vi "生成word报表.vi"(0 "Array输入":refnum<vi>, 1 "产品序号":string, 2 "标注图":T1(plugin-control), 3 "Array输入 2":refnum<vi>, 4 "测试人":string, 5 "部位":string, 8 "反射图":T1(plugin-control) caption="Original Image") -> (14 "报告生成路径":path)   [LabVIEW 2018]
uses:
  <vilib>/Utility/NIReport.llb/Report Type.ctl
  <vilib>/Utility/NIReport.llb/Append Report Text (str wrap).vi
  <vilib>/addons/_office/word.llb/Word Edit Cell ([dbl]).vi
  <vilib>/addons/_office/word.llb/Word Edit Cell (str).vi
  <vilib>/Utility/NIReport.llb/Append Report Text (num wrap).vi
  <vilib>/Utility/NIReport.llb/NI_report.lvclass
  <vilib>/addons/_office/NI_ReportGenerationToolkit.lvlib
  <vilib>/Utility/NIReport.llb/Word/NI_Word.lvclass
  <vilib>/Utility/NIReport.llb/NI_ReportGenerationCore.lvlib
  <vilib>/addons/_office/word.llb/Word Edit Cell ([str]).vi
panel:
  out "分层累计缺陷占比":dbl
  out "分层Z值":dbl[](array[numeric])
  out "缺陷个数 2":i32
  out "分层数据":dbl[][](array[numeric])
  out "弥散累计缺陷占比":dbl
  out "弥散数据":dbl[][](array[numeric])
  out "弥散Z值":dbl[](array[numeric])
  out "缺陷个数":i32
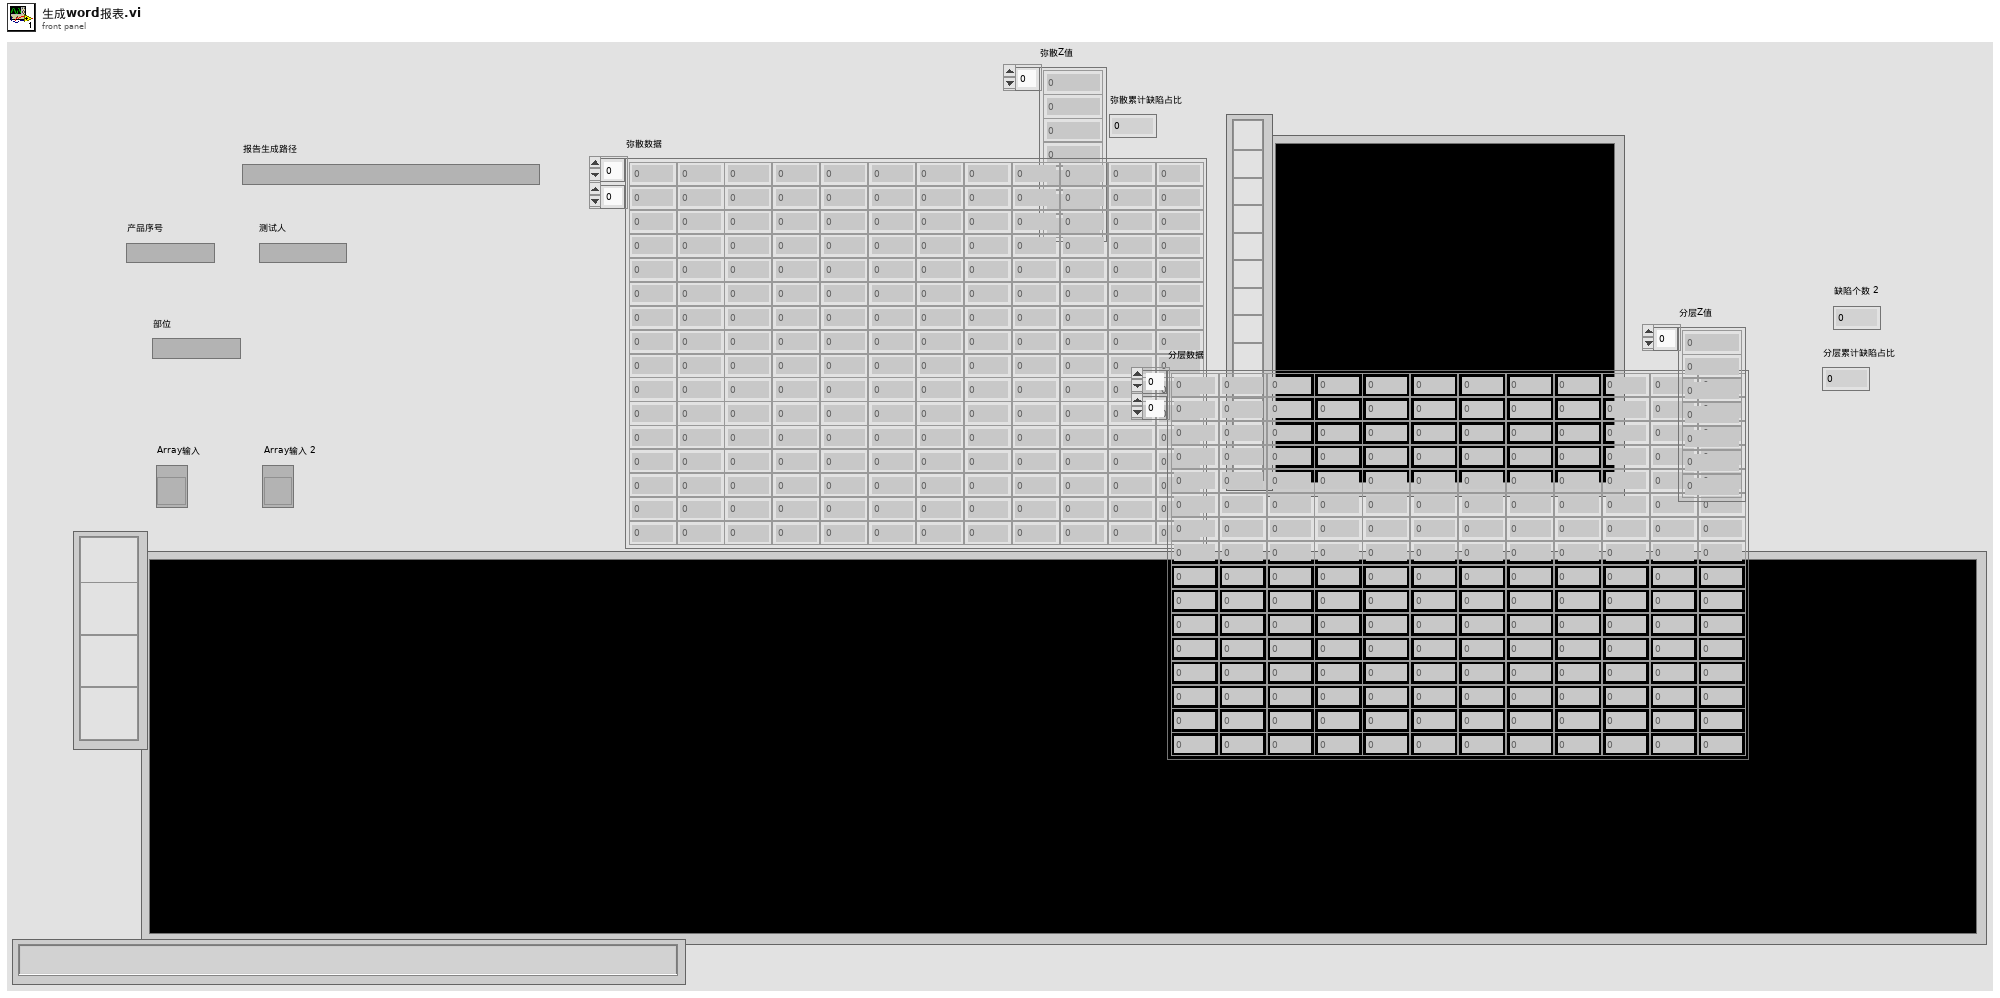
[diagram p1: front panel]
types:
  T1 = typedef "IMAQ Image.ctl" = refnum<image>
  T2 = cluster{"position (Excel)":cluster{"row":i32, "column":i32}, "name (Excel)":string, "bookmark (Word)":string}
  T3 = typedef "NI_ReportGenerationCore.lvlib/Report Type.ctl" = enum16{"HTML", "Word", "Excel"}
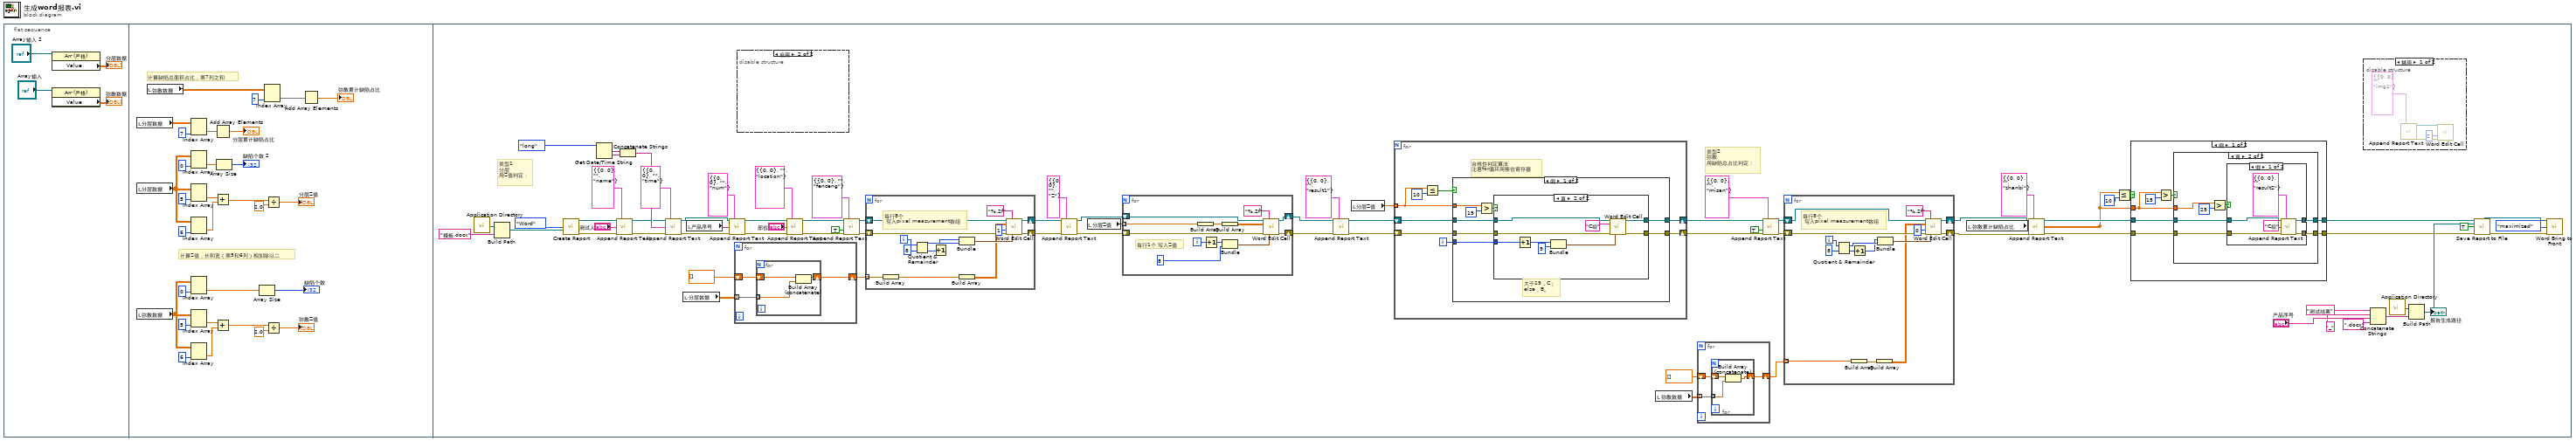
[diagram p0: block diagram]
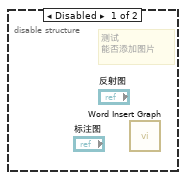
[diagram p3: hidden frame]
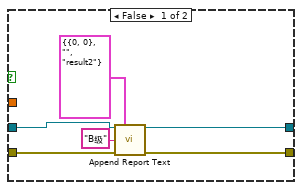
[diagram p4: hidden frame]
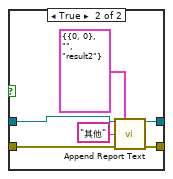
[diagram p5: hidden frame]
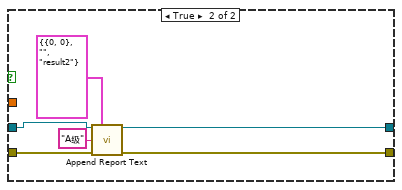
[diagram p6: hidden frame]
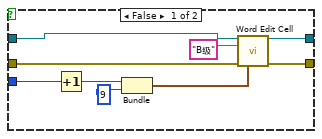
[diagram p7: hidden frame]
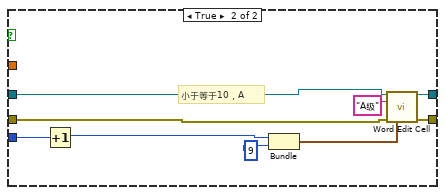
[diagram p8: hidden frame]
diagram:
  n1 = flat-sequence {
    frame #0 {
      n2 = property class="Arr (严格)"(reference="Array输入 2") -> ("Value"=→"分层数据":dbl[][])  [unwired: 1 in, 2 out]
      n3 = property class="Arr (严格)"(reference="Array输入") -> ("Value"=→"弥散数据":dbl[][])  [unwired: 1 in, 2 out]
    }
    frame #1 {
      # "计算缺陷总面积占比，第7列之和"
      # "计算Z值，长和宽（第5和6列）相加除以二"
      n4 = local read "分层数据"() -> (w8:dbl[][])
      n5 = local read "分层数据"() -> (w19:dbl[][])
      n6 = local read "弥散数据"() -> (w34:dbl[][])
      n7 = local read "弥散数据"() -> (w23:dbl[][])
      n8 = Index Array(array=w8, index (col)=7 ("禁用的索引 (列)")) -> (element=w6:dbl[])  [unwired: 1 in]
      n9 = Index Array(array=w19, index (col)=0 ("禁用的索引 (列)")) -> (element=w16:dbl[])  [unwired: 1 in]
      n10 = Index Array(array=w19, index (col)=5 ("索引")) -> (element=w13:dbl[])  [unwired: 1 in]
      n11 = Index Array(array=w19, index (col)=6 ("索引")) -> (element=w14:dbl[])  [unwired: 1 in]
      n12 = Index Array(array=w34, index (col)=0 ("禁用的索引 (列)")) -> (element=w31:dbl[])  [unwired: 1 in]
      n13 = Index Array(array=w34, index (col)=5 ("索引")) -> (element=w28:dbl[])  [unwired: 1 in]
      n14 = Index Array(array=w34, index (col)=6 ("索引")) -> (element=w29:dbl[])  [unwired: 1 in]
      n15 = Add Array Elements(numeric array=w6) -> (sum=→"分层累计缺陷占比":dbl)
      n16 = Add(x=w13, y=w14) -> (x+y=w15:dbl[])
      n17 = Add(x=w28, y=w29) -> (x+y=w30:dbl[])
      n18 = Array Size(array=w16) -> (size(s)=→"缺陷个数 2":i32)
      n19 = Array Size(array=w31) -> (size(s)=→"缺陷个数":i32)
      n20 = Index Array(array=w23, index (col)=7 ("禁用的索引 (列)")) -> (element=w21:dbl[])  [unwired: 1 in]
      n21 = Divide(x=w15, y=2.0) -> (x/y=→"分层Z值":dbl[])
      n22 = Divide(x=w30, y=2.0) -> (x/y=→"弥散Z值":dbl[])
      n23 = Add Array Elements(numeric array=w21) -> (sum=→"弥散累计缺陷占比":dbl)
    }
    frame #2 {
      # "类型2\n弥散\n用缺陷总占比判定："
      # "类型1\n分层\n用Z值判定："
      n24 = call <vilib>:"Application Directory.vi"() -> ("Application Directory"=w90:path)
      n25 = Build Path(base path=w90, name or relative path="模板.docx") -> (appended path=w89:path)
      n26 = call <vilib>:"Create Report.vi"("report type"=Report_Type."Word" ("Report Type"), "template (empty)"=w89) -> ("report out"=w82:refnum<class "NI_report.lvclass">, "error out"=w79:errorcluster)  [unwired: 12 in]
      n27 = Get Date/Time String(date format (0)=enum16{"short", "long", "abbreviated"}."long" ("日期格式(0)")) -> (date string=w88:string, time string=w86:string)  [unwired: 2 in]
      n28 = call-poly <vilib>:"Append Report Text.vi"("report in"=w82, "MS Office parameters"=T2 {"position (Excel)"={"row"=0, "column"=0}, "name (Excel)"="", "bookmark (Word)"="name"}, "text"="测试人", "error in (no error)"=w79) -> ("report out"=w81:refnum<class "NI_report.lvclass">, "error out"=w80:errorcluster)  [unwired: 8 in, 2 out]
      n29 = Concatenate Strings(w88, w86) -> (w87:string)
      n30 = call-poly <vilib>:"Append Report Text.vi"("report in"=w81, "MS Office parameters"=T2 {"position (Excel)"={"row"=0, "column"=0}, "name (Excel)"="", "bookmark (Word)"="time"}, "text"=w87, "error in (no error)"=w80) -> ("report out"=w85:refnum<class "NI_report.lvclass">, "error out"=w84:errorcluster)  [unwired: 8 in, 2 out]
      n31 = local read "分层数据"() -> (w93:dbl[][])
      n32 = local read "产品序号"() -> (w56:string)
      n33 = call-poly <vilib>:"Append Report Text.vi"("report in"=w85, "MS Office parameters"=T2 {"position (Excel)"={"row"=0, "column"=0}, "name (Excel)"="", "bookmark (Word)"="num"}, "text"=w56, "error in (no error)"=w84) -> ("report out"=w58:refnum<class "NI_report.lvclass">, "error out"=w57:errorcluster)  [unwired: 8 in, 2 out]
      n34 = for {
        tunnel: w93 -> [w229] mode=indexing
        shift-right: [w227] -> w83
        shift-left: dbl[] [] ("元素") -> [w228]
        n35 = for {
          tunnel: w229 -> [w232] mode=indexing
          shift-right: [w230] -> w227
          shift-left: w228 -> [w231]
          n36 = Build Array (concatenate)(w231, w232) -> (w230:dbl[])
        }
      }
      n37 = disable-structure shown="启用" {
        frame Disabled {
          # "测试\n能否添加图片"
          n38 = call <vilib>:"Word Insert Graph.vi"() -> ()  [unwired: 12 in, 4 out]
        }
        frame Enabled {
        }
      }
      n39 = call-poly <vilib>:"Append Report Text.vi"("report in"=w58, "MS Office parameters"=T2 {"position (Excel)"={"row"=0, "column"=0}, "name (Excel)"="", "bookmark (Word)"="location"}, "text"="部位", "error in (no error)"=w57) -> ("report out"=w60:refnum<class "NI_report.lvclass">, "error out"=w59:errorcluster)  [unwired: 8 in, 2 out]
      n40 = call-poly <vilib>:"Append Report Text.vi"("report in"=w60, "MS Office parameters"=T2 {"position (Excel)"={"row"=0, "column"=0}, "name (Excel)"="", "bookmark (Word)"="fenceng"}, "append on new line? (F)"=TRUE, "error in (no error)"=w59) -> ("report out"=w92:refnum<class "NI_report.lvclass">, "error out"=w91:errorcluster)  [unwired: 8 in, 2 out]
      n41 = for {
        shift-right: [w247] -> w77
        shift-left: w92 -> [w242]
        shift-right: [w246] -> w108
        shift-left: w91 -> [w241]
        tunnel: w83 -> [w235] mode=indexing
        i -> [w243]
        # "每行8个\n 写入pixel measurement数组"
        n42 = Build Array(w235) -> (w237:dbl[])
        n43 = Quotient & Remainder(x=w243, y=8) -> (x-y*floor(x/y)=w240:i32, floor(x/y)=w239:i32)
        n44 = Increment(x=w239) -> (x+1=w238:i32)
        n45 = Bundle(w238, w240) -> (w245:cluster{i32, i32})  [unwired: 1 in]
        n46 = Build Array(w237) -> (w236:dbl[][])
        n47 = call-poly <vilib>:"Word Edit Cell.vi"("report in"=w242, "format string (%.3f)"="%.2f", "value"=w236, "table index (-1)"=i16 1, "error in (no error)"=w241, "start (0, 0)"=w245) -> ("report out"=w247:refnum<class "NI_report.lvclass">, "error out"=w246:errorcluster)  [unwired: 8 in]
      }
      n48 = call-poly <vilib>:"Append Report Text.vi"("report in"=w77, "MS Office parameters"=T2 {"position (Excel)"={"row"=0, "column"=0}, "name (Excel)"="", "bookmark (Word)"="Z"}, "error in (no error)"=w108) -> ("report out"=w101:refnum<class "NI_report.lvclass">, "error out"=w100:errorcluster)  [unwired: 9 in, 2 out]
      n49 = local read "分层Z值"() -> (w94:dbl[])
      n50 = for {
        shift-right: [w226] -> w97
        shift-left: w101 -> [w223]
        shift-right: [w225] -> w96
        shift-left: w100 -> [w222]
        tunnel: w94 -> [w218] mode=indexing
        i -> [w216]
        # "每行1个 写入Z值"
        n51 = Build Array(w218) -> (w220:dbl[])
        n52 = Increment(x=w216) -> (x+1=w221:i32)
        n53 = Build Array(w220) -> (w219:dbl[][])
        n54 = Bundle(w221, "y"=8) -> (w224:cluster{i32, "y":i32})  [unwired: 1 in]
        n55 = call-poly <vilib>:"Word Edit Cell.vi"("report in"=w223, "format string (%.3f)"="%.2f", "value"=w219, "error in (no error)"=w222, "start (0, 0)"=w224) -> ("report out"=w226:refnum<class "NI_report.lvclass">, "error out"=w225:errorcluster)  [unwired: 9 in]
      }
      n56 = call-poly <vilib>:"Append Report Text.vi"("report in"=w97, "MS Office parameters"=T2 {"position (Excel)"={"row"=0, "column"=0}, "name (Excel)"="", "bookmark (Word)"="result1"}, "error in (no error)"=w96) -> ("report out"=w98:refnum<class "NI_report.lvclass">, "error out"=w99:errorcluster)  [unwired: 9 in, 2 out]
      n57 = local read "分层Z值"() -> (w95:dbl[])
      n58 = for {
        shift-right: [w173] -> w53
        shift-left: w98 -> [w176]
        shift-right: [w174] -> w52
        shift-left: w99 -> [w175]
        tunnel: w95 -> [w172] mode=indexing
        i -> [w177]
        # "合格性判定算法\n注意for循环用移位寄存器"
        n59 = Less Or Equal?(x=w172, y=10) -> (x <= y?=w178:bool)
        n60 = case shown="假" w178 {
          tunnel: w177 -> [w184 w212]
          tunnel: w176 -> [w183 w211]
          tunnel: w175 -> [w182 w210]
          tunnel: [w180 w209] -> w174
          tunnel: [w181 w208] -> w173
          tunnel: w172 -> [w187 _]
          frame False {
            # "大于19，C；\nelse，B。"
            n61 = Greater?(x=w187, y=19) -> (0:w185:bool)
            n62 = case shown="真" w185 {
              tunnel: w184 -> [w188 w201]
              tunnel: w183 -> [w192 w200]
              tunnel: w182 -> [w191 w199]
              tunnel: [w190 w198] -> w181
              tunnel: [w189 w197] -> w180
              frame False {
                n63 = Increment(x=w188) -> (x+1=w196:i32)
                n64 = Bundle(w196, "y"=9) -> (w195:cluster{i32, "y":i32})  [unwired: 1 in]
                n65 = call-poly <vilib>:"Word Edit Cell.vi"("report in"=w192, "value"="B级", "error in (no error)"=w191, "start (0, 0)"=w195) -> ("report out"=w190:refnum<class "NI_report.lvclass">, "error out"=w189:errorcluster)  [unwired: 10 in]
              }
              frame True {
                n66 = Increment(x=w201) -> (x+1=w205:i32)
                n67 = Bundle(w205, "y"=9) -> (w204:cluster{i32, "y":i32})  [unwired: 1 in]
                n68 = call-poly <vilib>:"Word Edit Cell.vi"("report in"=w200, "value"="C级", "error in (no error)"=w199, "start (0, 0)"=w204) -> ("report out"=w198:refnum<class "NI_report.lvclass">, "error out"=w197:errorcluster)  [unwired: 10 in]
              }
            }
          }
          frame True {
            # "小于等于10，A"
            n69 = Increment(x=w212) -> (x+1=w214:i32)
            n70 = Bundle(w214, "y"=9) -> (w206:cluster{i32, "y":i32})  [unwired: 1 in]
            n71 = call-poly <vilib>:"Word Edit Cell.vi"("report in"=w211, "value"="A级", "error in (no error)"=w210, "start (0, 0)"=w206) -> ("report out"=w208:refnum<class "NI_report.lvclass">, "error out"=w209:errorcluster)  [unwired: 10 in]
          }
        }
      }
      n72 = local read "弥散数据"() -> (w51:dbl[][])
      n73 = for {
        tunnel: w51 -> [w168] mode=indexing
        shift-right: [w166] -> w47
        shift-left: dbl[] [] ("元素") -> [w167]
        n74 = for {
          tunnel: w168 -> [w171] mode=indexing
          shift-right: [w169] -> w166
          shift-left: w167 -> [w170]
          n75 = Build Array (concatenate)(w170, w171) -> (w169:dbl[])
        }
      }
      n76 = call-poly <vilib>:"Append Report Text.vi"("report in"=w53, "MS Office parameters"=T2 {"position (Excel)"={"row"=0, "column"=0}, "name (Excel)"="", "bookmark (Word)"="misan"}, "append on new line? (F)"=TRUE, "error in (no error)"=w52) -> ("report out"=w49:refnum<class "NI_report.lvclass">, "error out"=w48:errorcluster)  [unwired: 8 in, 2 out]
      n77 = for {
        shift-right: [w165] -> w45
        shift-left: w49 -> [w160]
        shift-right: [w164] -> w44
        shift-left: w48 -> [w159]
        tunnel: w47 -> [w153] mode=indexing
        i -> [w161]
        # "每行8个\n 写入pixel measurement数组"
        n78 = Quotient & Remainder(x=w161, y=8) -> (x-y*floor(x/y)=w158:i32, floor(x/y)=w157:i32)
        n79 = Build Array(w153) -> (w155:dbl[])
        n80 = Increment(x=w157) -> (x+1=w156:i32)
        n81 = Build Array(w155) -> (w154:dbl[][])
        n82 = Bundle(w156, w158) -> (w163:cluster{i32, i32})  [unwired: 1 in]
        n83 = call-poly <vilib>:"Word Edit Cell.vi"("report in"=w160, "format string (%.3f)"="%.2f", "value"=w154, "table index (-1)"=i16 0, "error in (no error)"=w159, "start (0, 0)"=w163) -> ("report out"=w165:refnum<class "NI_report.lvclass">, "error out"=w164:errorcluster)  [unwired: 8 in]
      }
      n84 = local read "弥散累计缺陷占比"() -> (w39:dbl)
      n85 = call-poly <vilib>:"Append Report Text.vi"("report in"=w45, "MS Office parameters"=T2 {"position (Excel)"={"row"=0, "column"=0}, "name (Excel)"="", "bookmark (Word)"="zhanbi"}, "text"=w39, "error in (no error)"=w44) -> ("report out"=w43:refnum<class "NI_report.lvclass">, "error out"=w42:errorcluster)  [unwired: 8 in, 2 out]
      n86 = Less Or Equal?(x=w39, y=10) -> (x <= y?=w40:bool)
      n87 = case shown="假" w40 {
        tunnel: w43 -> [w117 w148]
        tunnel: w42 -> [w115 w147]
        tunnel: [w114 w146] -> w35
        tunnel: [w116 w145] -> w36
        tunnel: w39 -> [w113 _]
        frame False {
          n88 = Greater?(x=w113, y=15) -> (0:w118:bool)
          n89 = case shown="真" w118 {
            tunnel: w117 -> [w123 w129]
            tunnel: [w122 w126] -> w116
            tunnel: w115 -> [w121 w128]
            tunnel: [w120 w127] -> w114
            tunnel: w113 -> [_ w131]
            frame False {
              n90 = call-poly <vilib>:"Append Report Text.vi"("report in"=w123, "MS Office parameters"=T2 {"position (Excel)"={"row"=0, "column"=0}, "name (Excel)"="", "bookmark (Word)"="result2"}, "text"="B级", "error in (no error)"=w121) -> ("report out"=w122:refnum<class "NI_report.lvclass">, "error out"=w120:errorcluster)  [unwired: 8 in, 2 out]
            }
            frame True {
              n91 = Greater?(x=w131, y=25) -> (0:w130:bool)
              n92 = case shown="假" w130 {
                tunnel: w129 -> [w136 w142]
                tunnel: w128 -> [w135 w141]
                tunnel: [w134 w140] -> w127
                tunnel: [w133 w139] -> w126
                frame False {
                  n93 = call-poly <vilib>:"Append Report Text.vi"("report in"=w136, "MS Office parameters"=T2 {"position (Excel)"={"row"=0, "column"=0}, "name (Excel)"="", "bookmark (Word)"="result2"}, "text"="C级", "error in (no error)"=w135) -> ("report out"=w133:refnum<class "NI_report.lvclass">, "error out"=w134:errorcluster)  [unwired: 8 in, 2 out]
                }
                frame True {
                  n94 = call-poly <vilib>:"Append Report Text.vi"("report in"=w142, "MS Office parameters"=T2 {"position (Excel)"={"row"=0, "column"=0}, "name (Excel)"="", "bookmark (Word)"="result2"}, "text"="其他", "error in (no error)"=w141) -> ("report out"=w139:refnum<class "NI_report.lvclass">, "error out"=w140:errorcluster)  [unwired: 8 in, 2 out]
                }
              }
            }
          }
        }
        frame True {
          n95 = call-poly <vilib>:"Append Report Text.vi"("report in"=w148, "MS Office parameters"=T2 {"position (Excel)"={"row"=0, "column"=0}, "name (Excel)"="", "bookmark (Word)"="result2"}, "text"="A级", "error in (no error)"=w147) -> ("report out"=w145:refnum<class "NI_report.lvclass">, "error out"=w146:errorcluster)  [unwired: 8 in, 2 out]
        }
      }
      n96 = disable-structure shown="禁用" {
        frame Disabled {
          n97 = call-poly <vilib>:"Append Report Text.vi"("MS Office parameters"=T2 {"position (Excel)"={"row"=0, "column"=0}, "name (Excel)"="", "bookmark (Word)"="img1"}) -> ("report out"=w111:refnum<class "NI_report.lvclass">, "error out"=w110:errorcluster)  [unwired: 11 in, 2 out]
          n98 = call-poly <vilib>:"Word Edit Cell.vi"("report in"=w111, "table index (-1)"=i16 2, "error in (no error)"=w110) -> ()  [unwired: 11 in, 2 out]
        }
        frame Enabled {
        }
      }
      n99 = Concatenate Strings("测试结果" ("字符串"), "_" ("名称或相对路径"), "产品序号", ".docx" ("名称或相对路径")) -> (w105:string)
      n100 = call <vilib>:"Application Directory.vi"() -> ("Application Directory"=w106:path)
      n101 = Build Path(base path=w106, name or relative path=w105) -> (appended path=w107:path)
      "报告生成路径" <- w107
      n102 = call-dynamic "Save Report to File.vi"("report in"=w36, "report file path"=w107, "prompt to replace? (F)"=TRUE, "error in (no error)"=w35) -> ("report out"=w104:refnum<class "NI_report.lvclass">, "error out"=w103:errorcluster)  [unwired: 10 in]
      n103 = call <vilib>:"Word Bring to Front.vi"("report in"=w104, "window state (maximized)"=enum16{"maximized", "minimized", "normal"}."maximized", "error in (no error)"=w103) -> ()  [unwired: 11 in, 2 out]
    }
  }
